vi "Write Menu Queue.vi"(8 "error in (no error)":errorcluster, 10 "Actor Framework.lvlib:Message Enqueuer":refnum<class "Message Enqueuer.lvclass">, 11 "Interface with menu in":refnum<class "Interface with menu.lvclass">) -> (0 "error out":errorcluster, 3 "Interface with menu out":refnum<class "Interface with menu.lvclass">)   [LabVIEW 2015, in "Interface with menu.lvclass"]
uses:
  Interface with menu.lvclass
  <vilib>/ActorFramework/Message Enqueuer/Message Enqueuer.lvclass
  Interface with menu.lvclass/Interface with menu.ctl
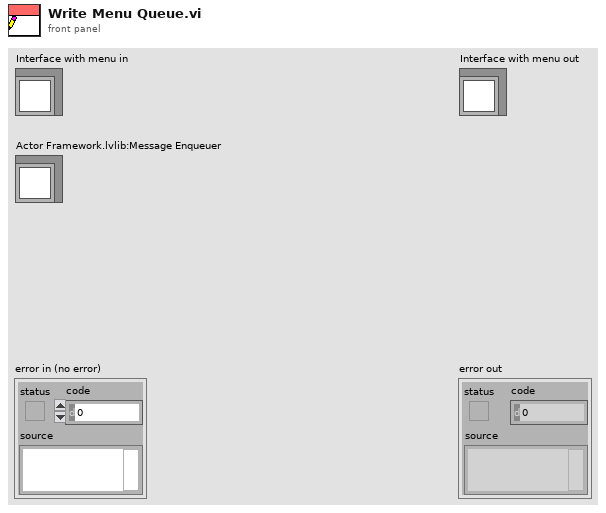
[diagram p1: front panel]
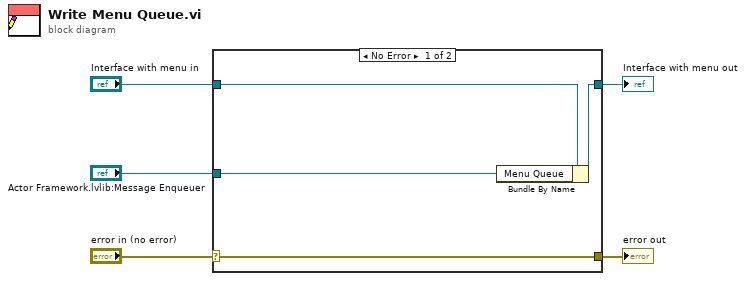
[diagram p0: block diagram]
diagram:
  n1 = case shown="No Error" "error in (no error)" {
    selector: "error in (no error)" -> [w9 w10]
    tunnel: [w9 w10] -> w4
    tunnel: [w7 w11] -> w2
    tunnel: "Interface with menu in" -> [w8 w11]
    tunnel: "Actor Framework.lvlib:Message Enqueuer" -> [w6 _]
    frame No Error {
      n2 = Bundle By Name(cluster=w8, "Menu Queue"=w6) -> (w7:refnum<class "Interface with menu.lvclass">)
    }
    frame Error {
    }
  }
  "error out" <- w4
  "Interface with menu out" <- w2
